vi "dfd_NStage MRate Response without Overall.vi"(5 "type (FLP)":enum16{"FLP", "FXP"}(ring), 6 "fs [Hz]":dbl, 7 "# freq bins (auto)":i32, 8 "error in (no error)":errorcluster, 9 "magnitude":u16(ring) items=["Linear", "dB", "Zero phase"], 10 "phase view":T1, 11 "multirate filters in":T2[](array[typedef]) {"mMRate_SumWl" min=1 max=32 step=1; "mMRate_InputIwl" min=1 max=32 step=1; "mMRate_GainWl" min=1 max=32 step=1; "mMRate_OutputWl" min=1 max=32 step=1; "mMRate_InputWl" min=1 max=32 step=1; "mMRate_CoefWl" min=1 max=32 step=1; "mMRate_Mode" items=["Default"=-1, "No Rate Change"=0, "Interpolation"=1, "Decimation"=2, "Interpolated"=3, "Rational"=4]}) -> (0 "error out":errorcluster, 2 "phase":cluster{dbl, "df":dbl, "phase":dbl[]}[](array[cluster]), 3 "mag":cluster{dbl, "df":dbl, "magnitude":dbl[]}[](array[cluster]))   [LabVIEW 2017, in "NI_DigFilterLicensed.lvlib"]
uses:
  <vilib>/addons/Digital Filter Design/NI_DigFilterLicensed.lvlib
  <vilib>/addons/Digital Filter Design/_Objects.llb/DFD Multirate Filter Obj.ctl
  <vilib>/addons/Digital Filter Design/_Objects.llb/DFD Multirate Mode.ctl
  <vilib>/addons/Digital Filter Design/_Objects.llb/DFD Coef Norm Type.ctl
  <vilib>/addons/Digital Filter Design/_Objects.llb/DFD Round-off Mode.ctl
  <vilib>/addons/Digital Filter Design/_Objects.llb/DFD FXP MRate Multiply Mode.ctl
  <vilib>/addons/Digital Filter Design/_Objects.llb/DFD Phase Setting.ctl
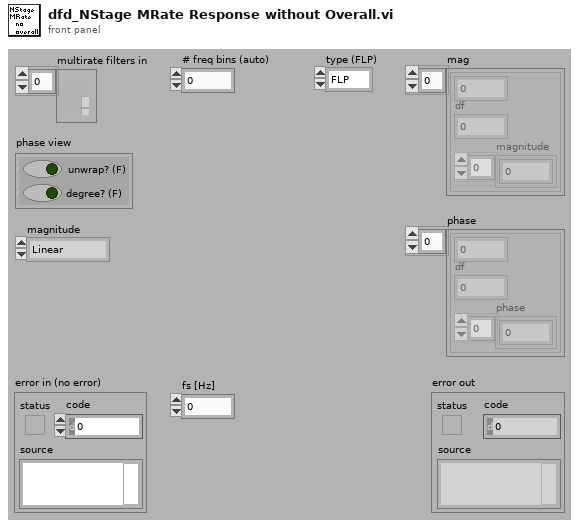
[diagram p1: front panel]
types:
  T1 = typedef "NI_DigFilterLicensed.lvlib/DFD Phase Setting.ctl" = cluster{"unwrap? (F)":bool, "degree? (F)":bool}
  T2 = typedef "NI_DigFilterLicensed.lvlib/DFD Multirate Filter Obj.ctl" = cluster{"mMRate_Structure":enum16{"CIC", "FIR", "IIR", "Lattice"}, "mMRate_Mode":T3, "mMRate_Factor":i32, "mMRate_FIRParams":cluster{"mMRate_FIR_H":dbl[], "mMRate_FIR_IsNyquist?":bool, "mMRate_FIR_IsSymmetric?":bool}, "mMRate_CICParams":cluster{"mMRate_CIC_#Stage":i32, "mMRate_CIC_Lag":i32, "mMRate_CIC_Type":enum16{"Lowpass", "Highpass"}}, "mMRate_Order":i32, "mMRate_Version":string, "mMRate_Comments":string, "mMRate_RationalFactor":cluster{"mMRate_L":i32, "mMRate_M":i32}, "mMRate_Fs":dbl, "mMRate_Quantized?":bool, "mMRate_QFilterGain":dbl, "mMRate_CoefWl":i16, "mMRate_Scaling":cluster{"mMRate_ScaleByPowerOf2?":bool, "mMRate_ScaleType":T4}, "mMRate_InputWl":i16, "mMRate_OutputWl":i16, "mMRate_OutputMode":T5, "mMRate_MultMode":T6, "mMRate_BitPruning":bool, "mMRate_GainWl":i16, "mMRate_OutputFwl":i16, "mMRate_SumIwl":i16, "mMRate_InputIwl ":i16, "mMRate_SumWl":i16, "mMRate_CoefIwl":i16}
  T3 = typedef "NI_DigFilterLicensed.lvlib/DFD Multirate Mode.ctl" = i16
  T4 = typedef "NI_DigFilterLicensed.lvlib/DFD Coef Norm Type.ctl" = enum16{"No Norm", "Time Domain 1-Norm", "Time Domain 2-Norm", "Time Domain Inf-Norm"}
  T5 = typedef "NI_DigFilterLicensed.lvlib/DFD Round-off Mode.ctl" = enum16{"Nearest", "Truncation"}
  T6 = typedef "NI_DigFilterLicensed.lvlib/DFD FXP MRate Multiply Mode.ctl" = enum16{"Truncated", "Full"}
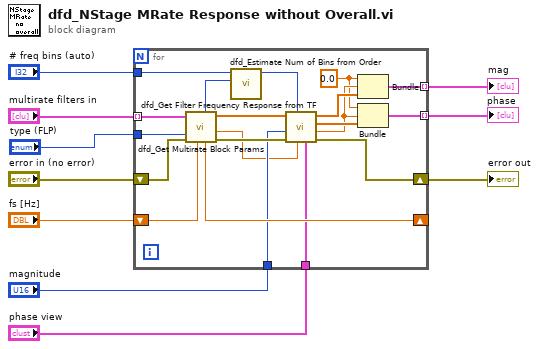
[diagram p0: block diagram]
diagram:
  n1 = for {
    shift-right: [w27] -> _
    shift-left: "fs [Hz]" -> [w28]
    shift-right: [w13] -> w6
    shift-left: "error in (no error)" -> [w29]
    tunnel: "multirate filters in" -> [w30] mode=indexing
    tunnel: "magnitude" -> [w22]
    tunnel: "phase view" -> [w21]
    tunnel: [w15] -> w4 mode=indexing
    tunnel: [w14] -> w5 mode=indexing
    tunnel: "# freq bins (auto)" -> [w12]
    tunnel: "type (FLP)" -> [w11]
    w16 = 0.0
    n2 = call <vilib>:"dfd_Get Multirate Block Params.vi"("fs in [Hz]"=w28, "error in (no error)"=w29, "type (FLP)"=w11, "multirate filter in"=w30) -> ("error out"=w25:errorcluster, "filter fs"=w20:dbl, "fs out [Hz]"=w27:dbl, "order"=w26:i32, "FIR"=w24:dbl[])  [unwired: 3 out]
    n3 = call <vilib>:"dfd_Estimate Num of Bins from Order.vi"("order"=w26, "# freq bins in"=w12) -> ("# freq bins out"=w23:i32)  [unwired: 9 out]
    n4 = call <vilib>:"dfd_Get Filter Frequency Response from TF.vi"("phase view"=w21, "fs [Hz]"=w20, "# freq bins (512)"=w23, "error in (no error)"=w25, "magnitude"=w22, "num"=w24) -> ("error out"=w13:errorcluster, "df"=w17:dbl, "phase"=w19:dbl[], "magnitude"=w18:dbl[])  [unwired: 1 in, 1 out]
    n5 = Bundle(w16, "df"=w17, "magnitude"=w18) -> (w15:cluster{dbl, "df":dbl, "magnitude":dbl[]})  [unwired: 1 out]
    n6 = Bundle(w16, "df"=w17, "phase"=w19) -> (w14:cluster{dbl, "df":dbl, "phase":dbl[]})  [unwired: 1 out]
  }
  "error out" <- w6
  "phase" <- w5
  "mag" <- w4
